vi "Read Multi-Point [MP] Core.vi"(8 "error in (no error)":errorcluster, 9 "array size":i32, 10 "maximum time (5s)":dbl[unit]=5000.0 caption="maximum time (5000 ms)", 11 "CS++DMM in":refnum<class "CS++DMM.lvclass">) -> (0 "error out":errorcluster, 1 "actual number of points":i32, 2 "reading array":dbl[](array[numeric]) format="%^.2e", 3 "CS++DMM out":refnum<class "CS++DMM.lvclass">)   [LabVIEW 2016, in "CS++DMM.lvlib" / "CS++DMM.lvclass"]
doc: "This VI initiates the measurement, waits for the DMM to return to the Idle state, and returns an array of measured values. The number of measurements the DMM takes is determined by the values you specify for the Trigger Count and Sample Count parameters of the IviDmm Configure Multi-Point [MP] VI.\n\nThis VI applies default values to properties that have not been set by the user under the following conditions:\n\n(1) If the user has not set the value of any property in the IviDmmMultiPoint extension group, the VI sets the IviDmm>>Multi-Point Acquisition>>Sample Count [MP] and IviDmm>>Multi-Point Acquisition>>Trigger Count [MP] properties to 1.\n\n(2) If the user has not set the value of the IviDmm>Measurement Operation Options>Auto Zero [AZ] property, the VI sets the value of this property to IVIDMM_VAL_AUTO_ZERO_OFF (0). \n\nNotes:\n\n(1) This VI is part of the IviDmmMultiPoint [MP] extension group.\n\n(2) After this VI executes, each element in the Reading Array parameter is an actual reading or a value indicating that an over-range condition occurred.\n\n(3) If an over-range condition occurs, the corresponding Reading Array element contains an IEEE defined NaN (Not a Number) value and the VI returns the IVIDMM_WARN_OVER_RANGE (0x3FFA2001) warning code. \n\n(4) You can test each element in the Reading Array parameter for an over-range condition by calling the IviDmm Is Over-Range VI.\n\n(5) This VI performs interchangeability checking when the IviDmm>>Inherent IVI Settings>>User Options>>Interchange Check property is set to TRUE. If the IviDmm>>Inherent IVI Settings>>User Options>>Spy property is set to TRUE, you use the NI Spy utility to view interchangeability warnings. You use the IviDmm Get Next Interchange Warning VI to retrieve interchangeability warnings when the IviDmm>>Inherent IVI Settings>>User Options>>Spy property is set to FALSE. For more information about interchangeability checking, refer to the help text for the IviDmm>>Inherent IVI Settings>>User Options>>Interchange Check property.\n\n(6) The class driver initiates an array of simulated measurements when this VI is called and the IviDmm>>Inherent IVI Settings>>User Options>>Simulate property is set to TRUE and the IviDmm>>Inherent IVI Settings>>User Options>>Use Specific Simulation property is set to FALSE. For information on how to configure a simulated measurement, refer to the online help manual."
uses:
  CS++DMM.lvclass
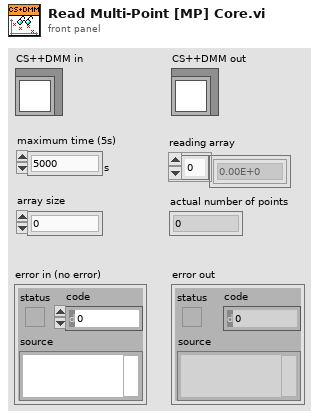
[diagram p1: front panel]
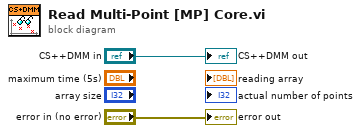
[diagram p0: block diagram]
diagram:
  "error out" <- "error in (no error)"
  "CS++DMM out" <- "CS++DMM in"
